vi "Write UUT_Info.vi"(8 "error in":errorcluster, 10 "UUT_Info":bool, 11 "Base Software in":refnum<class "Base Software.lvclass">) -> (0 "error out":errorcluster, 3 "Base Software out":refnum<class "Base Software.lvclass">)   [LabVIEW 2019, in "Base Software.lvlib" / "Main.lvlib" / "Base Software.lvclass"]
uses:
  Project/Base Software.lvclass
  Project/Base Software.lvclass/Base Software.ctl
  builds/Engine/Engine.lvlibp/Custom Controls/System Status.ctl
  Indicators/Write Model.vi
  Indicators/Write Serial.vi
  builds/Engine/Engine.lvlibp/Project/Engine.lvclass
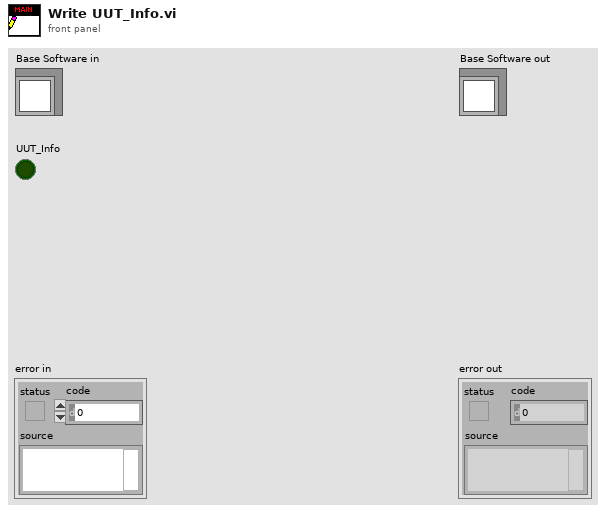
[diagram p1: front panel]
types:
  T1 = typedef "Engine.lvlibp/Engine.lvclass/System Status.ctl" = enum16{"Logged Off", "UUT_Info_Missing", "Idle", "Error", "Warning", "Loading", "Config", "Manual", "Automation", "Report_View", "Previous"}
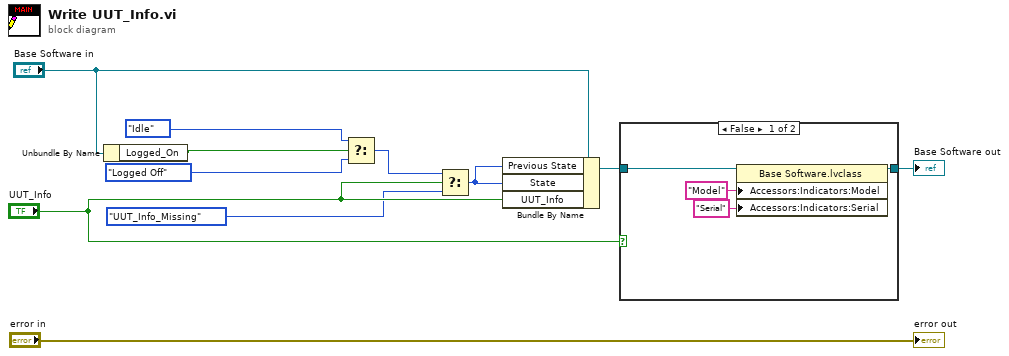
[diagram p0: block diagram]
diagram:
  n1 = Unbundle By Name("Base Software in") -> ("Logged_On"=w6:bool)
  n2 = Select(t=System_Status."Idle" ("State"), s=w6, f=System_Status."Logged Off" ("State")) -> (s? t:f=w8:T1)
  n3 = Select(t=w8, s="UUT_Info", f=System_Status."UUT_Info_Missing" ("State")) -> (s? t:f=w4:T1)
  n4 = Bundle By Name(cluster="Base Software in", "Previous State"=w4, "State"=w4, "UUT_Info"="UUT_Info") -> (w10:refnum<class "Base Software.lvclass">)
  n5 = case shown="False" "UUT_Info" {
    tunnel: w10 -> [w15 w16]
    tunnel: [w14 w16] -> w9
    frame False {
      n6 = property class="Base Software.lvclass"(reference=w15, "Accessors:Indicators:Model"="Model" ("Model"), "Accessors:Indicators:Serial"="Serial" ("Serial")) -> (reference out=w14:refnum<class "Base Software.lvclass">)  [unwired: 1 in, 1 out]
    }
    frame True {
    }
  }
  "Base Software out" <- w9
  "error out" <- "error in"
